vi "Write Systems.vi"(8 "error in":errorcluster, 10 "system":T1, 11 "SystemConfigRepo in":refnum<class "SystemConfigRepo.lvclass">) -> (0 "error out":errorcluster, 3 "SystemConfigRepo out":refnum<class "SystemConfigRepo.lvclass">)   [LabVIEW 2013, in "PL Framework Configuration Tool.lvlib" / "SystemConfigRepo.lvclass"]
uses:
  SystemConfigRepo.lvclass
  Framework Configuration Classes/platypus configuration/systems cluster.ctl
  Framework Configuration Classes/system configuration/PL_System Configuration.lvclass
  Framework Configuration Classes/platypus configuration/targets cluster.ctl
  Framework Configuration Classes/target configuration/PL_Target Configuration.lvclass
  Framework Configuration Classes/platypus configuration/engines cluster.ctl
  <vilib>/NI/Module Execution Interface/Engine Configuration/engine configuration.lvclass
  <vilib>/NI/Tag Bus Module Framework/module configuration/TBM module configuration.lvclass
  SystemConfigRepo.lvclass/SystemConfigRepo.ctl
  Framework Configuration Classes/platypus configuration/PLConfigurationSerializer.lvlib
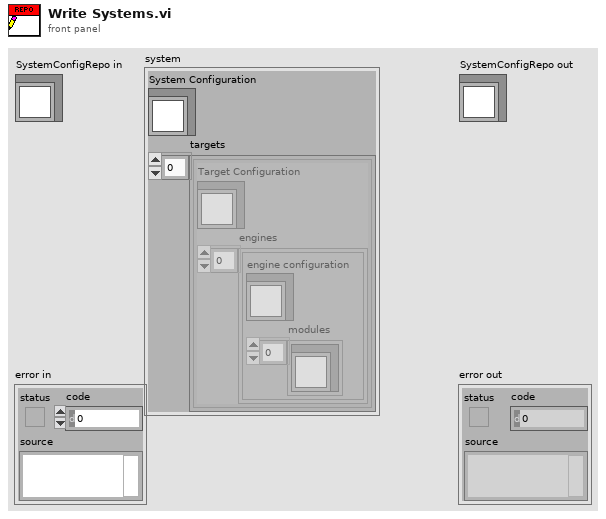
[diagram p1: front panel]
types:
  T1 = typedef "PLConfigurationSerializer.lvlib/systems cluster.ctl" = cluster{"System Configuration":refnum<class "PL_System Configuration.lvclass">, "targets":T2[]}
  T2 = typedef "PLConfigurationSerializer.lvlib/targets cluster.ctl" = cluster{"Target Configuration":refnum<class "PL_Target Configuration.lvclass">, "engines":T3[]}
  T3 = typedef "PLConfigurationSerializer.lvlib/engines cluster.ctl" = cluster{"engine configuration":refnum<class "engine configuration.lvclass">, "modules":refnum<class "TBM module configuration.lvclass">[]}
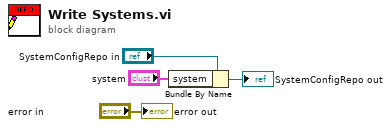
[diagram p0: block diagram]
diagram:
  n1 = Bundle By Name(cluster="SystemConfigRepo in", "system"="system") -> (→"SystemConfigRepo out":refnum<class "SystemConfigRepo.lvclass">)
  "error out" <- "error in"
